vi "final16.vi"() -> ()   [LabVIEW 2016]
uses:
  <vilib>/Analysis/NI_AALBase.lvlib
  <vilib>/Analysis/NI_AALPro.lvlib
  <vilib>/Instr/_visa.llb/VISA Configure Serial Port (Instr).vi
panel:
  out "Reading slope":dbl
  out "Reading intercept":dbl
  out "calculated noise":dbl[](array[numeric])
  out "Reads array":dbl[](array[numeric])
  out "calculated intercept":dbl
  out "calculated slope":dbl
  in  "Tab Control":T1(tab)
  in  "Choose saving file format":T2(ring)
  out "Gain tabs":enum32{"Gain 32", "Gain 64", "Gain 128"}(tab)
  out "intercept_gain32":dbl
  out "slope_gain32":dbl
  out "intercept_gain64":dbl
  out "slope_gain64":dbl
  out "intercept_gain128":dbl
  out "slope_gain128":dbl
  out "Setting offset":bool
  in  "Gain":u16(ring) items=["32", "64", "128"]
  in  "Function":u16(ring) items=["Read data ", "Compare different gains", "Execute calibration"]
  in  "Start operation":bool
  in  "Cycles":dbl min=1.0 step=1.0
  in  "Stop":bool
  out "String passed to Arduino":string
  out "Mean":dbl format="%0.2f"
  out "Variance":dbl format="%0.2f"
  out "Standard deviation":dbl format="%0.2f"
  out "Received data":string[](array[string])
  out "Setting variables":bool
  out "Conversion [g]":dbl
  out "PoliBa Logo":picture
  out "Standard deviation [g]":dbl
  out "Variance [g2]":dbl
  out "Absolute error":dbl
  out "Relative error":dbl
  out "Writing to EEPROM":bool
  out "Calibration - read data":dbl[][](array[numeric])
  out "Noise_gain32":dbl[](array[numeric])
  out "Absolute errors array":dbl[](array[numeric])
  out "Relative errors array":dbl[](array[numeric])
  out "Noise_gain64":dbl[](array[numeric])
  out "Noise_gain128":dbl[](array[numeric])
  out "XY Graph":cluster{"Weights":dbl[], "Measures":dbl[]}(graph)
  in  "Anti-panic":enum32{"Not here", "Maybe here"}(tab)
  out "Debug array":string[](array[string])
  out "Received data array":dbl[](array[numeric])
  out "Read offsets":dbl[](array[numeric])
  # "Select all options, then press \"Start operation\" button"
  # "Calibration"
  # "Nerd zone"
  # "Don't panic!\n\nKeep your towel with you!"
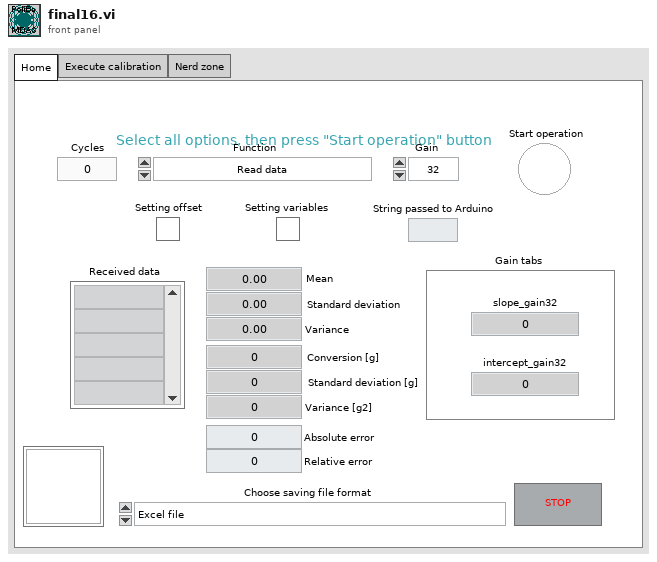
[diagram p1: front panel]
types:
  T1 = enum32{"Home", "Execute calibration", "Nerd zone"}
  T2 = enum16{"Excel file", "Tab separated values", "Text file"}
  T3 = typedef "imagedata.ctl" = cluster{"image type":i32, "image depth":i32, "image":u8[], "mask":u8[], "colors":u32[], "Rectangle":cluster{"left":i16, "top":i16, "right":i16, "bottom":i16}}
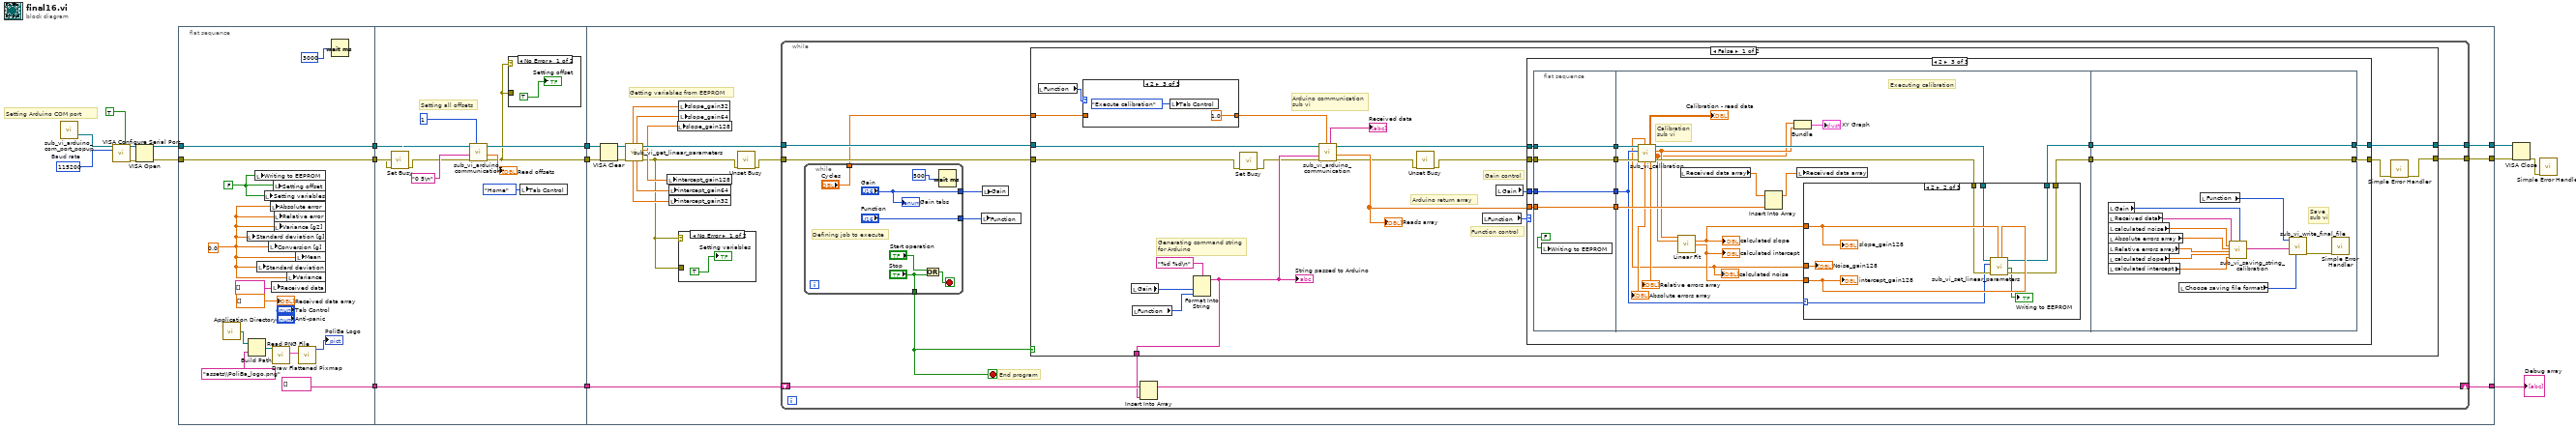
[diagram p0: block diagram]
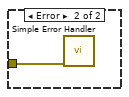
[diagram p2: hidden frame]
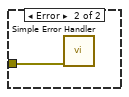
[diagram p3: hidden frame]
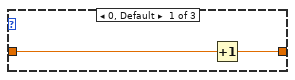
[diagram p4: hidden frame]
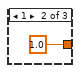
[diagram p5: hidden frame]
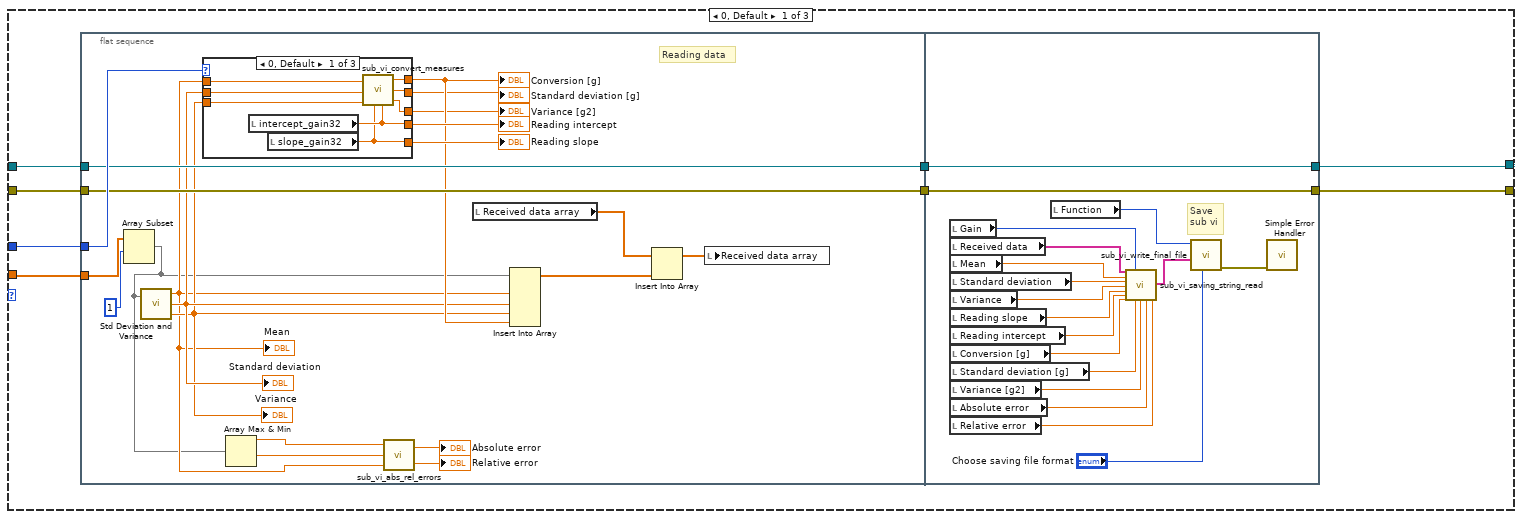
[diagram p6: hidden frame]
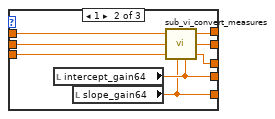
[diagram p7: hidden frame]
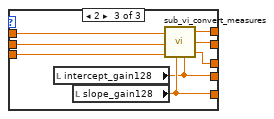
[diagram p8: hidden frame]
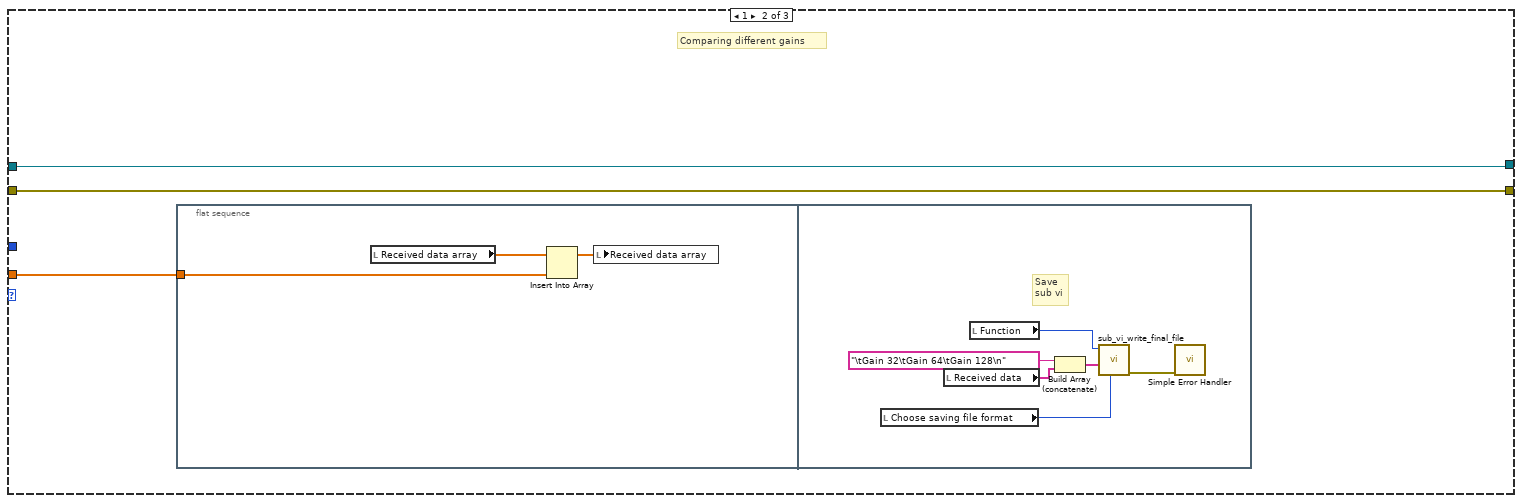
[diagram p9: hidden frame]
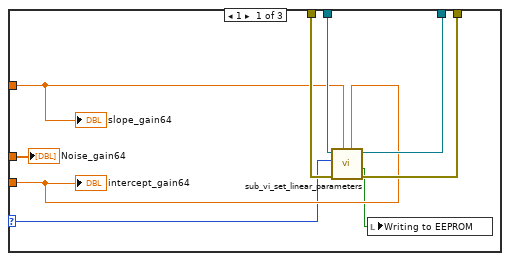
[diagram p10: hidden frame]
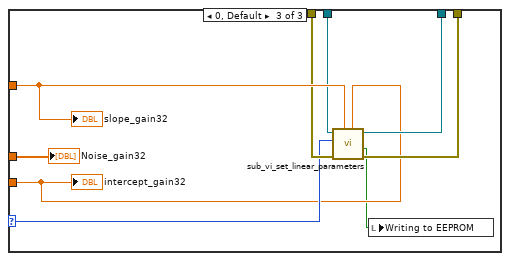
[diagram p11: hidden frame]
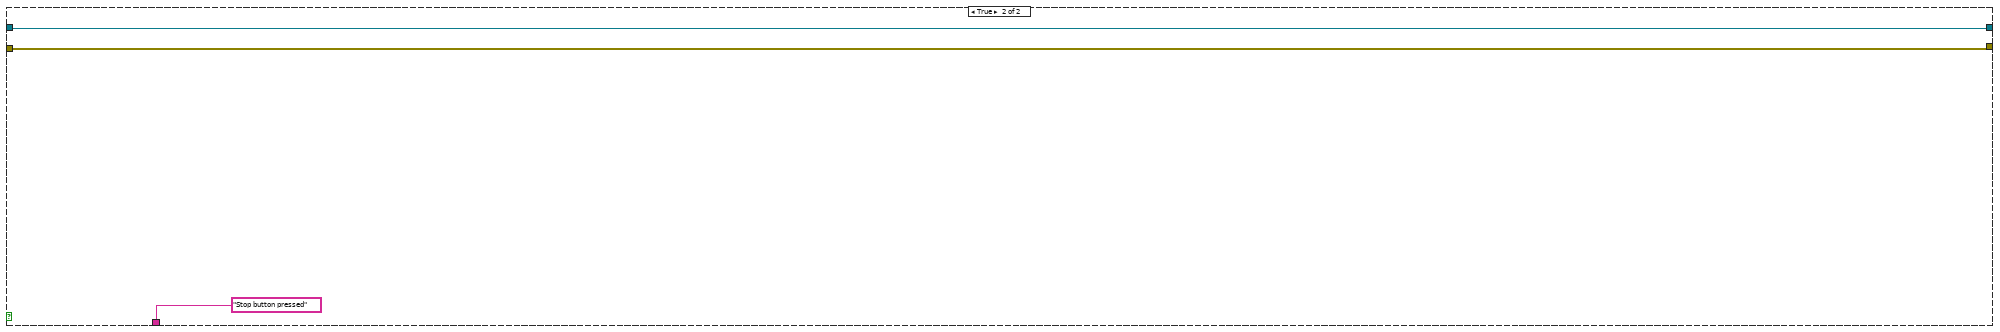
[diagram p12: hidden frame]
diagram:
  w17 = u32 115200  # Baud rate
  # "Setting Arduino COM port"
  n1 = call "sub_vi_arduino_com_port_popup.vi"() -> ("Arduino COM port 2"=w7:refnum<visa-resource-name>)  [unwired: 19 in]
  n2 = call-poly "VISA Configure Serial Port"("VISA resource name"=w7, "Enable Termination\nChar (T)"=TRUE ("Enable Termination\nChar (T)"), "baud rate (9600)"=w17) -> ("VISA resource name out"=w15:refnum<visa-resource-name>, "error out"=w16:errorcluster)  [unwired: 11 in]
  n3 = VISA Open(error in (no error)=w16, VISA resource name=w15) -> (VISA resource name=w12:refnum<visa-resource-name>, error out=w13:errorcluster)  [unwired: 3 in]
  n4 = flat-sequence {
    tunnel: w12 -> [w29]
    tunnel: w13 -> [w30]
    tunnel: [w30] -> w6
    tunnel: [w29] -> w4
    tunnel: [string[] []] -> w1
    tunnel: w6 -> [w35]
    tunnel: [w32] -> w5
    tunnel: w4 -> [w40]
    tunnel: [w39] -> w3
    tunnel: [w33] -> w2
    tunnel: w1 -> [w33]
    tunnel: [w57] -> w11
    tunnel: [w56] -> w9
    tunnel: [w55] -> w8
    tunnel: w5 -> [w59]
    tunnel: w3 -> [w58]
    tunnel: w2 -> [w47]
    frame #0 {
      w19 = FALSE ("Setting offset")
      w18 = 0.0 ("Standard deviation")
      n5 = call <vilib>:"Application Directory.vi"() -> ("Application Directory"=w22:path)
      n6 = local write "Standard deviation [g]"(w18) -> ()
      n7 = Build Path(base path=w22, name or relative path="assets\\PoliBa_logo.png") -> (appended path=w20:path)
      n8 = local write "Writing to EEPROM"(w19) -> ()
      n9 = local write "Standard deviation"(w18) -> ()
      n10 = local write "Setting variables"(w19) -> ()
      n11 = local write "Conversion [g]"(w18) -> ()
      n12 = local write "Absolute error"(w18) -> ()
      n13 = local write "Received data"(string[] []) -> ()
      n14 = call <vilib>:"Read PNG File.vi"("path to PNG file"=w20) -> ("image data"=w24:T3)  [unwired: 8 in, 2 out]
      n15 = local write "Setting offset"(w19) -> ()
      n16 = local write "Relative error"(w18) -> ()
      n17 = local write "Variance [g2]"(w18) -> ()
      n18 = local write "Variance"(w18) -> ()
      n19 = local write "Mean"(w18) -> ()
      n20 = call <vilib>:"Draw Flattened Pixmap.vi"("image data"=w24) -> ("new picture"=→"PoliBa Logo":picture)  [unwired: 8 in]
      n21 = Wait (ms)(milliseconds to wait=u32 3000) -> ()  [unwired: 1 out]
      "Received data array" <- dbl[] []
    }
    frame #1 {
      # "Setting all offsets"
      n22 = call <vilib>:"Set Busy.vi"("error in (no error)"=w35) -> ("error out"=w34:errorcluster)  [unwired: 9 in, 1 out]
      n23 = call "sub_vi_arduino_communication.vi"("Cycles"=1, "error in (no error)"=w34, "write buffer"="0 5\n", "VISA resource name in"=w40) -> ("error out"=w32:errorcluster, "Reads array"=→"Read offsets":dbl[], "VISA resource name out"=w39:refnum<visa-resource-name>)  [unwired: 2 in, 1 out]
      n24 = case shown="No Error" w32 {
        tunnel: w32 -> [_ w42]
        frame No Error {
          "Setting offset" <- TRUE ("Setting offset")
        }
        frame Error {
          n25 = call <vilib>:"Simple Error Handler.vi"("error in (no error)"=w42) -> ()  [unwired: 4 in, 5 out]
        }
      }
      n26 = local write "Tab Control"(T1."Home" ("Tab Control")) -> ()
    }
    frame #2 {
      # "Getting variables from EEPROM"
      n27 = VISA Clear(VISA resource name=w58, error in (no error)=w59) -> (VISA resource name out=w52:refnum<visa-resource-name>, error out=w50:errorcluster)
      n28 = call "sub_vi_get_linear_parameters.vi"("error in"=w50, "VISA resource name in"=w52) -> ("error out"=w43:errorcluster, "intercept_2"=w49:dbl, "slope_2"=w46:dbl, "VISA resource name out"=w51:refnum<visa-resource-name>, "intercept_1"=w54:dbl, "slope_1"=w45:dbl, "intercept_0"=w53:dbl, "slope_0"=w44:dbl)  [unwired: 2 in]
      n29 = local write "intercept_gain128"(w49) -> ()
      n30 = local write "intercept_gain64"(w54) -> ()
      n31 = local write "intercept_gain32"(w53) -> ()
      n32 = local write "slope_gain128"(w46) -> ()
      n33 = local write "slope_gain32"(w44) -> ()
      n34 = local write "slope_gain64"(w45) -> ()
      n35 = case shown="No Error" w43 {
        tunnel: w43 -> [_ w61]
        frame No Error {
          "Setting variables" <- TRUE ("Setting offset")
        }
        frame Error {
          n36 = call <vilib>:"Simple Error Handler.vi"("error in (no error)"=w61) -> ()  [unwired: 4 in, 5 out]
        }
      }
      n37 = call <vilib>:"Unset Busy.vi"("error in (no error)"=w43) -> ("error out"=w48:errorcluster)  [unwired: 10 in]
      n38 = while {
        tunnel: w48 -> [w67]
        tunnel: w51 -> [w68]
        shift-right: [w72] -> w57
        shift-left: w47 -> [w71]
        tunnel: [w70] -> w56
        tunnel: [w69] -> w55
        stop <- w64 stop-if-true
        # "End program"
        n39 = while {
          tunnel: ["Function"] -> w62
          tunnel: ["Gain"] -> w63
          tunnel: ["Cycles"] -> w65
          tunnel: ["Stop"] -> w64
          stop <- w75 stop-if-true
          # "Defining job to execute"
          n40 = Or(x="Start operation", y="Stop") -> (x .or. y?=w75:bool)
          n41 = Wait (ms)(milliseconds to wait=u32 500) -> ()  [unwired: 1 out]
          "Gain tabs" <- "Gain"
        }
        n42 = local write "Function"(w62) -> ()
        n43 = local write "Gain"(w63) -> ()
        n44 = case shown="False" w64 {
          tunnel: [w91 w265] -> w70
          tunnel: [w98 w266] -> w69
          tunnel: w68 -> [w97 w266]
          tunnel: w67 -> [w83 w265]
          tunnel: [w93 "Stop button pressed"] -> w66
          tunnel: w65 -> [w81 _]
          frame False {
            # "Generating command string\nfor Arduino"
            # "Function control"
            # "Arduino return array"
            # "Gain control"
            # "Arduino communication\nsub vi"
            n45 = local read "Function"() -> (w82:u16)
            n46 = case shown="2" w82 {
              tunnel: w81 -> [w100 _ _]
              tunnel: [w101 1.0 ("Cycles") 1.0 ("Cycles")] -> w80
              frame 0, Default {
                n47 = Increment(x=w100) -> (x+1=w101:dbl)
              }
              frame 1 {
              }
              frame 2 {
                n48 = local write "Tab Control"(T1."Execute calibration" ("Tab Control")) -> ()
              }
            }
            n49 = local read "Gain"() -> (w89:u16)
            n50 = local read "Function"() -> (w90:u16)
            n51 = Format Into String(format string="%d %d\n", w89, w90) -> (resulting string=w93:string)  [unwired: 2 in, 1 out]
            "String passed to Arduino" <- w93
            n52 = call <vilib>:"Set Busy.vi"("error in (no error)"=w83) -> ("error out"=w84:errorcluster)  [unwired: 9 in, 1 out]
            n53 = call "sub_vi_arduino_communication.vi"("Cycles"=w80, "error in (no error)"=w84, "write buffer"=w93, "VISA resource name in"=w97) -> ("error out"=w86:errorcluster, "Reads array"=w95:dbl[], "VISA resource name out"=w96:refnum<visa-resource-name>, "Received data"=→"Received data":string[])  [unwired: 2 in]
            "Reads array" <- w95
            n54 = call <vilib>:"Unset Busy.vi"("error in (no error)"=w86) -> ("error out"=w85:errorcluster)  [unwired: 10 in]
            n55 = local read "Function"() -> (w87:u16)
            n56 = local read "Gain"() -> (w88:u16)
            n57 = case shown="2" w87 {
              tunnel: w88 -> [w111 _ w194]
              tunnel: w95 -> [w112 w176 w197]
              tunnel: w96 -> [w110 w178 w199]
              tunnel: w85 -> [w109 w177 w198]
              tunnel: [w108 w178 w196] -> w98
              tunnel: [w105 w177 w195] -> w92
              frame 0, Default {
                n58 = flat-sequence {
                  tunnel: w112 -> [w124]
                  tunnel: w111 -> [w132]
                  tunnel: w110 -> [w129]
                  tunnel: w109 -> [w128]
                  tunnel: [w129] -> w107
                  tunnel: [w128] -> w106
                  tunnel: [w173] -> w108
                  tunnel: w107 -> [w173]
                  tunnel: w106 -> [w172]
                  tunnel: [w172] -> w105
                  frame #0 {
                    # "Reading data"
                    n59 = Array Subset(array=w124, index=1) -> (w117:dbl[])  [unwired: 1 in]
                    n60 = call <vilib>:"Std Deviation and Variance.vi"("X"=w117) -> ("mean"=w118:dbl, "standard deviation"=w120:dbl, "variance"=w119:dbl)  [unwired: 1 in]
                    "Standard deviation" <- w120
                    "Variance" <- w119
                    "Mean" <- w118
                    n61 = case shown="0, Default" w132 {
                      tunnel: [w141 w149 w157] -> w125
                      tunnel: w118 -> [w136 w144 w152]
                      tunnel: [w137 w147 w154] -> w126
                      tunnel: [w138 w148 w153] -> w127
                      tunnel: [w140 w146 w156] -> w122
                      tunnel: [w139 w145 w155] -> w121
                      tunnel: w120 -> [w135 w143 w151]
                      tunnel: w119 -> [w134 w142 w150]
                      frame 0, Default {
                        n62 = local read "intercept_gain32"() -> (w138:dbl)
                        n63 = local read "slope_gain32"() -> (w137:dbl)
                        n64 = call "sub_vi_convert_measures.vi"("Mean"=w136, "Standard deviation"=w135, "Variance"=w134, "Slope"=w137, "Intercept"=w138) -> ("Converted mean"=w141:dbl, "Converted std deviation"=w140:dbl, "Converted variance"=w139:dbl)  [unwired: 2 in]
                      }
                      frame 1 {
                        n65 = local read "intercept_gain64"() -> (w148:dbl)
                        n66 = local read "slope_gain64"() -> (w147:dbl)
                        n67 = call "sub_vi_convert_measures.vi"("Mean"=w144, "Standard deviation"=w143, "Variance"=w142, "Slope"=w147, "Intercept"=w148) -> ("Converted mean"=w149:dbl, "Converted std deviation"=w146:dbl, "Converted variance"=w145:dbl)  [unwired: 2 in]
                      }
                      frame 2 {
                        n68 = local read "intercept_gain128"() -> (w153:dbl)
                        n69 = local read "slope_gain128"() -> (w154:dbl)
                        n70 = call "sub_vi_convert_measures.vi"("Mean"=w152, "Standard deviation"=w151, "Variance"=w150, "Slope"=w154, "Intercept"=w153) -> ("Converted mean"=w157:dbl, "Converted std deviation"=w156:dbl, "Converted variance"=w155:dbl)  [unwired: 2 in]
                      }
                    }
                    "Conversion [g]" <- w125
                    "Reading intercept" <- w127
                    "Reading slope" <- w126
                    "Standard deviation [g]" <- w122
                    "Variance [g2]" <- w121
                    n71 = Array Max & Min(array=w117) -> (max value=w115:dbl, min value=w116:dbl)  [unwired: 2 out]
                    n72 = call "sub_vi_abs_rel_errors.vi"("Measure"=w118, "Min"=w116, "Max"=w115) -> ("Relative error"=→"Relative error":dbl, "Absolute error"=→"Absolute error":dbl)
                    n73 = local read "Received data array"() -> (w133:dbl[])
                    n74 = Insert Into Array(array=w117, new element #1=w118, new element #2=w120, new element #3=w119, new element #4=w125) -> (w130:dbl[])  [unwired: 1 in]
                    n75 = Insert Into Array(array=w133, new element=w130) -> (w131:dbl[])  [unwired: 1 in]
                    n76 = local write "Received data array"(w131) -> ()
                  }
                  frame #1 {
                    # "Save\nsub vi"
                    n77 = local read "Gain"() -> (w160:u16)
                    n78 = local read "Received data"() -> (w170:string[])
                    n79 = local read "Mean"() -> (w169:dbl)
                    n80 = local read "Standard deviation"() -> (w168:dbl)
                    n81 = local read "Variance"() -> (w167:dbl)
                    n82 = local read "Reading slope"() -> (w164:dbl)
                    n83 = local read "Reading intercept"() -> (w166:dbl)
                    n84 = local read "Conversion [g]"() -> (w165:dbl)
                    n85 = local read "Standard deviation [g]"() -> (w162:dbl)
                    n86 = local read "Variance [g2]"() -> (w161:dbl)
                    n87 = local read "Absolute error"() -> (w159:dbl)
                    n88 = local read "Relative error"() -> (w158:dbl)
                    n89 = local read "Function"() -> (w175:u16)
                    n90 = call "sub_vi_saving_string_read.vi"("Received data"=w170, "Mean"=w169, "Standard deviation"=w168, "Variance"=w167, "Slope"=w164, "Intercept"=w166, "Conversion"=w165, "Gain"=w160, "Converted std dev"=w162, "Converted variance"=w161, "Abs error"=w159, "Relative error"=w158) -> ("Resulting string"=w171:string[])  [unwired: 15 in]
                    n91 = call "sub_vi_write_final_file.vi"("Extension"="Choose saving file format", "1D data"=w171, "Function"=w175) -> ("error out"=w174:errorcluster)  [unwired: 8 in]
                    n92 = call <vilib>:"Simple Error Handler.vi"("error in (no error)"=w174) -> ()  [unwired: 4 in, 5 out]
                  }
                }
              }
              frame 1 {
                # "Comparing different gains"
                n93 = flat-sequence {
                  tunnel: w176 -> [w181]
                  frame #0 {
                    n94 = local read "Received data array"() -> (w180:dbl[])
                    n95 = Insert Into Array(array=w180, new element=w181) -> (w179:dbl[])  [unwired: 1 in]
                    n96 = local write "Received data array"(w179) -> ()
                  }
                  frame #1 {
                    # "Save\nsub vi"
                    n97 = local read "Choose saving file format"() -> (w182:T2)
                    n98 = local read "Received data"() -> (w186:string[])
                    n99 = local read "Function"() -> (w183:u16)
                    n100 = Build Array (concatenate)("\tGain 32\tGain 64\tGain 128\n", w186) -> (w187:string[])
                    n101 = call "sub_vi_write_final_file.vi"("Extension"=w182, "1D data"=w187, "Function"=w183) -> ("error out"=w185:errorcluster)  [unwired: 8 in]
                    n102 = call <vilib>:"Simple Error Handler.vi"("error in (no error)"=w185) -> ()  [unwired: 4 in, 5 out]
                  }
                }
              }
              frame 2 {
                n103 = flat-sequence {
                  tunnel: w194 -> [w201]
                  tunnel: w197 -> [w202]
                  tunnel: w198 -> [w203]
                  tunnel: w199 -> [w204]
                  tunnel: [w204] -> w191
                  tunnel: [w203] -> w190
                  tunnel: [w202] -> w189
                  tunnel: [w201] -> w188
                  tunnel: [w213] -> w193
                  tunnel: [w211] -> w192
                  tunnel: w191 -> [w221]
                  tunnel: w190 -> [w220]
                  tunnel: w189 -> [w218]
                  tunnel: w188 -> [w210]
                  tunnel: [w262] -> w195
                  tunnel: [w263] -> w196
                  tunnel: w193 -> [w263]
                  tunnel: w192 -> [w262]
                  frame #0 {
                    n104 = local write "Writing to EEPROM"(FALSE ("Writing to EEPROM")) -> ()
                  }
                  frame #1 {
                    # "Calibration\nsub vi"
                    # "Executing calibration"
                    n105 = call "sub_vi_calibration.vi"("error in (no error)"=w220, "Gain"=w210, "VISA resource name"=w221) -> ("error out"=w212:errorcluster, "Weights"=w206:dbl[], "Measures"=w207:dbl[], "VISA resource name out"=w214:refnum<visa-resource-name>, "Relative errors array"=→"Relative errors array":dbl[], "Calibration - read data"=→"Calibration - read data":dbl[][], "Absolute errors array"=→"Absolute errors array":dbl[], "Noise"=w208:dbl[])  [unwired: 1 in]
                    "calculated noise" <- w208
                    n106 = call <vilib>:"Linear Fit.vi"("Y"=w207, "X"=w206) -> ("slope"=w223:dbl, "intercept"=w222:dbl)  [unwired: 9 in, 3 out]
                    "calculated slope" <- w223
                    "calculated intercept" <- w222
                    n107 = local read "Received data array"() -> (w219:dbl[])
                    n108 = Insert Into Array(array=w219, new element=w218) -> (w209:dbl[])  [unwired: 1 in]
                    n109 = Bundle("Weights"=w206, "Measures"=w207) -> (→"XY Graph":cluster{"Weights":dbl[], "Measures":dbl[]})  [unwired: 1 in]
                    n110 = local write "Received data array"(w209) -> ()
                    n111 = case shown="2" w210 {
                      selector: w210 -> [w226 w235 w245]
                      tunnel: w223 -> [w228 w241 w250]
                      tunnel: w222 -> [w227 w240 w244]
                      tunnel: w214 -> [w232 w239 w248]
                      tunnel: [w230 w237 w249] -> w213
                      tunnel: w212 -> [w231 w238 w247]
                      tunnel: [w229 w236 w246] -> w211
                      tunnel: w208 -> [w225 w234 w243]
                      frame 1 {
                        n112 = call "sub_vi_set_linear_parameters.vi"("intercept"=w227, "slope"=w228, "error in (no error)"=w231, "gain"=w226, "VISA resource name in"=w232) -> ("error out"=w229:errorcluster, "Writing to EEPROM"=w224:bool, "VISA resource name out"=w230:refnum<visa-resource-name>)  [unwired: 3 in, 1 out]
                        n113 = local write "Writing to EEPROM"(w224) -> ()
                        "slope_gain64" <- w228
                        "intercept_gain64" <- w227
                        "Noise_gain64" <- w225
                      }
                      frame 2 {
                        n114 = call "sub_vi_set_linear_parameters.vi"("intercept"=w240, "slope"=w241, "error in (no error)"=w238, "gain"=w235, "VISA resource name in"=w239) -> ("error out"=w236:errorcluster, "Writing to EEPROM"=→"Writing to EEPROM":bool, "VISA resource name out"=w237:refnum<visa-resource-name>)  [unwired: 3 in, 1 out]
                        "slope_gain128" <- w241
                        "intercept_gain128" <- w240
                        "Noise_gain128" <- w234
                      }
                      frame 0, Default {
                        n115 = call "sub_vi_set_linear_parameters.vi"("intercept"=w244, "slope"=w250, "error in (no error)"=w247, "gain"=w245, "VISA resource name in"=w248) -> ("error out"=w246:errorcluster, "Writing to EEPROM"=w242:bool, "VISA resource name out"=w249:refnum<visa-resource-name>)  [unwired: 3 in, 1 out]
                        n116 = local write "Writing to EEPROM"(w242) -> ()
                        "slope_gain32" <- w250
                        "intercept_gain32" <- w244
                        "Noise_gain32" <- w243
                      }
                    }
                  }
                  frame #2 {
                    # "Save\nsub vi"
                    n117 = local read "Gain"() -> (w251:u16)
                    n118 = local read "Received data"() -> (w258:string[])
                    n119 = local read "calculated noise"() -> (w257:dbl[])
                    n120 = local read "Absolute errors array"() -> (w256:dbl[])
                    n121 = local read "Relative errors array"() -> (w255:dbl[])
                    n122 = local read "calculated slope"() -> (w254:dbl)
                    n123 = local read "calculated intercept"() -> (w253:dbl)
                    n124 = local read "Choose saving file format"() -> (w252:T2)
                    n125 = local read "Function"() -> (w261:u16)
                    n126 = call "sub_vi_saving_string_calibration.vi"("Received data"=w258, "calculated noise"=w257, "Absolute errors array"=w256, "Relative errors array"=w255, "calculated slope"=w254, "calculated intercept"=w253, "gain"=w251) -> ("Resulting array"=w259:string[])  [unwired: 12 in]
                    n127 = call "sub_vi_write_final_file.vi"("Extension"=w252, "1D data"=w259, "Function"=w261) -> ("error out"=w260:errorcluster)  [unwired: 8 in]
                    n128 = call <vilib>:"Simple Error Handler.vi"("error in (no error)"=w260) -> ()  [unwired: 4 in, 5 out]
                  }
                }
              }
            }
            n129 = call <vilib>:"Simple Error Handler.vi"("error in (no error)"=w92) -> ("error out"=w91:errorcluster)  [unwired: 4 in, 4 out]
          }
          frame True {
          }
        }
        n130 = Insert Into Array(array=w71, new element=w66) -> (w72:string[])  [unwired: 1 in]
      }
    }
  }
  n131 = VISA Close(VISA resource name=w8, error in (no error)=w9) -> (error out=w10:errorcluster)
  n132 = call <vilib>:"Simple Error Handler.vi"("error in (no error)"=w10) -> ()  [unwired: 4 in, 5 out]
  "Debug array" <- w11
